vi "ВП relative Error calc.vi"(1 "X":dbl, 2 "Xk":dbl, 3 "d":dbl, 4 "C":dbl) -> (0 "Относительная погрешность, %":dbl)   [LabVIEW 2013]
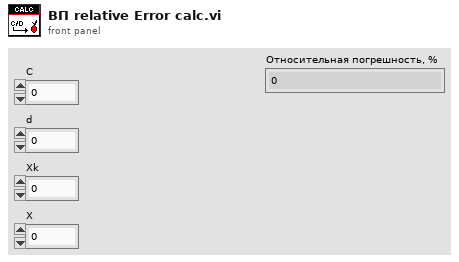
[diagram p1: front panel]
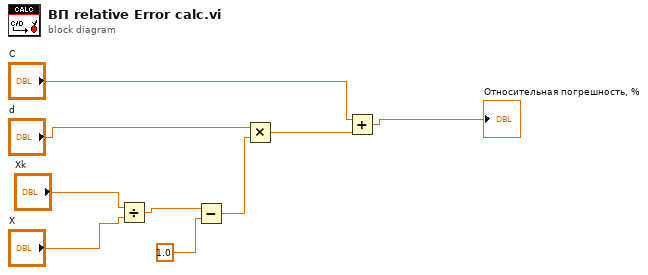
[diagram p0: block diagram]
diagram:
  n1 = Divide(x="Xk", y="X") -> (x/y=w7:dbl)
  n2 = Subtract(x=w7, y=1.0) -> (x-y=w4:dbl)
  n3 = Multiply(x="d", y=w4) -> (x*y=w3:dbl)
  n4 = Add(x="C", y=w3) -> (x+y=→"Относительная погрешность, %":dbl)
